vi "Main.vi"() -> ()   [LabVIEW 2020]
doc: "Use this template to build a simple state machine design pattern. Each state executes code and determines which state to transition to."
uses:
  controls/StateMachineVariables.ctl
  <vilib>/vision/Avi.llb/IMAQ AVI2 Refnum.ctl
  <vilib>/userDefined/High Color/IMAQdx.ctl
  <vilib>/vision/Deep Learning.llb/IMAQ DL Model Refnum.ctl
  <vilib>/vision/Image Controls.llb/IMAQ Image.ctl
  controls/State.ctl
panel:
  in  "Cluster":T1
  in  "Turn on the replay mode":bool=TRUE
  out "Replay mode":bool
  in  "?":T6(tab)
  in  "Camera Name":refnum<k21> caption="IMAQdx Session"
  out "fps cam":dbl
  out "height":u32
  out "width":u32
  in  "Start Frame Number":u32
  out "Actual frame":u32
  in  "Frame increment":i32=1
  in  "Video fps":u32=30
  in  "Video filename":string="test_moving2.avi"
  in  "Height":i32=1080
  in  "Width":i32=1920
  out "fps detection":dbl
  out "Distance":sgl(graph)
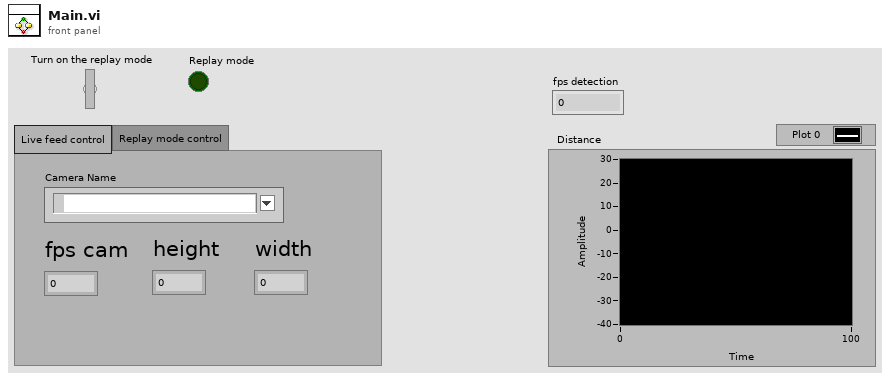
[diagram p1: front panel]
types:
  T1 = typedef "StateMachineVariables.ctl" = cluster{"AVI Refnum":T2, "Session ID":T3, "TensorFlow model refnum":T4, "Image refnum":T5, "VI path":path, "Horizontal distance":dbl, "Lateral distance":dbl, "Relative speed":dbl, "FPS":dbl}
  T2 = typedef "IMAQ AVI2 Refnum.ctl" = refnum<k20>
  T3 = typedef "IMAQdx.ctl" = refnum<k21>
  T4 = typedef "IMAQ DL Model Refnum.ctl" = refnum<k20>
  T5 = typedef "IMAQ Image.ctl" = refnum<image>
  T6 = enum32{"Live feed control", "Replay mode control"}
  T7 = typedef "State.ctl" = enum16{"Initialize VI path", "Initialize Video Session", "Initialize Cam session", "Initialize TensorFlow Model", "Initialize Image refnum", "Get video frame", "Get Cam frame", "Analyze image", "Update reaction space"}
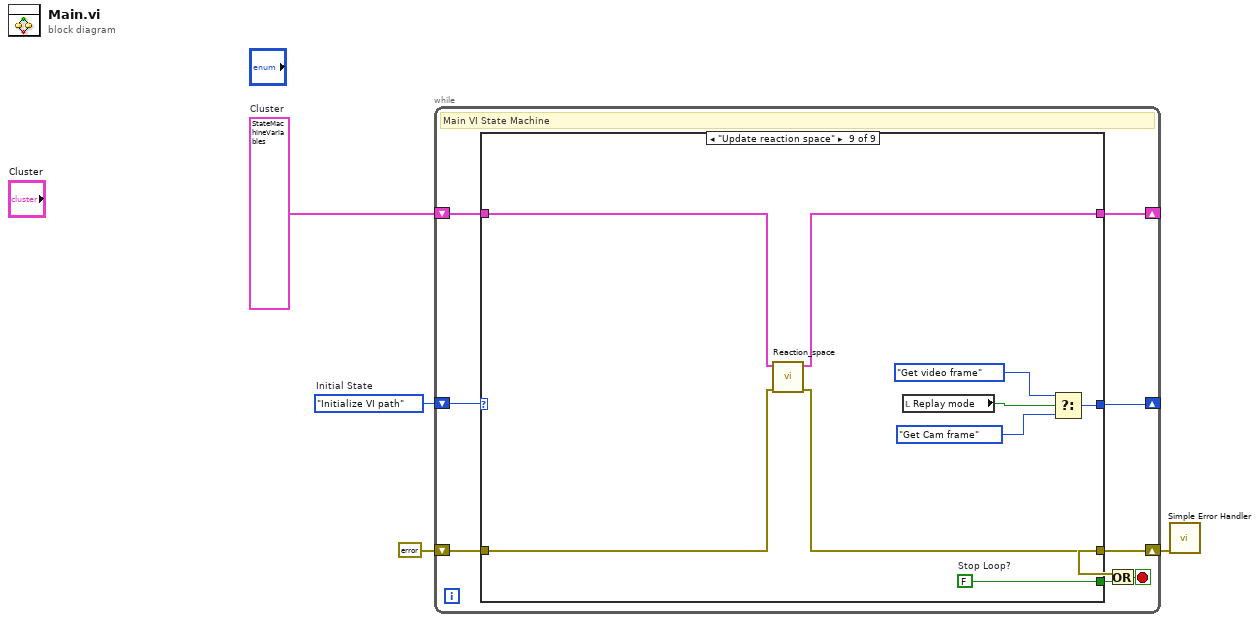
[diagram p0: block diagram]
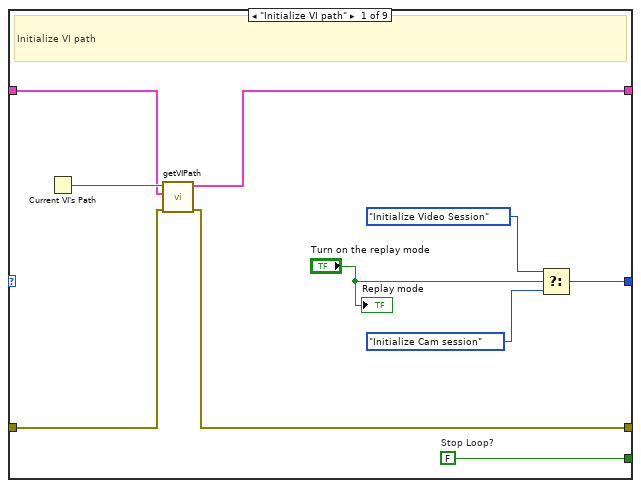
[diagram p2: hidden frame]
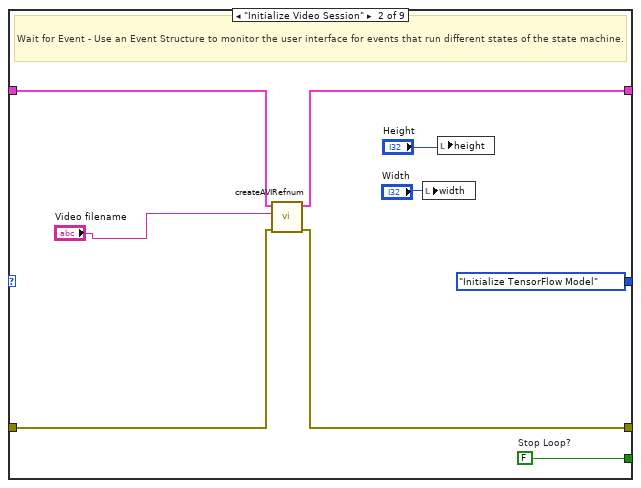
[diagram p3: hidden frame]
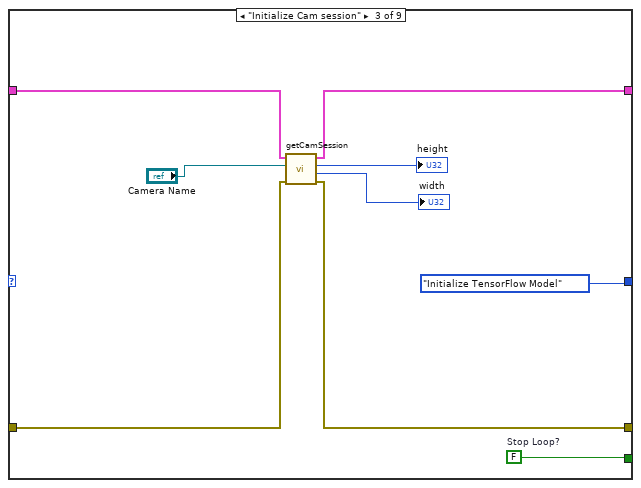
[diagram p4: hidden frame]
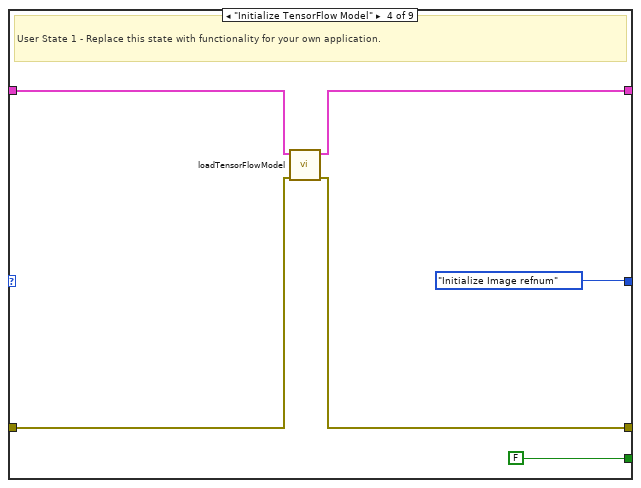
[diagram p5: hidden frame]
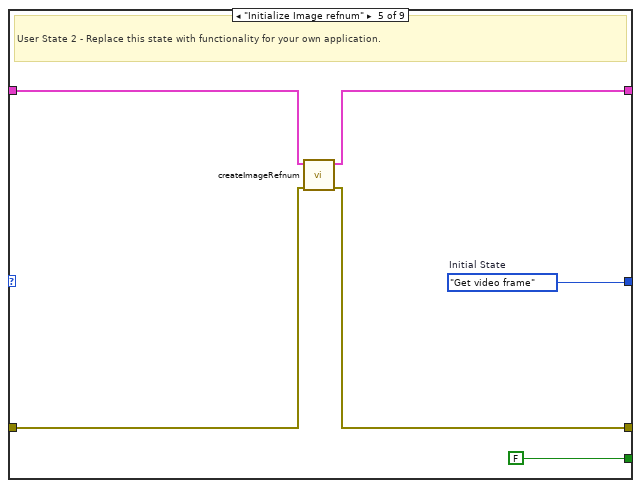
[diagram p6: hidden frame]
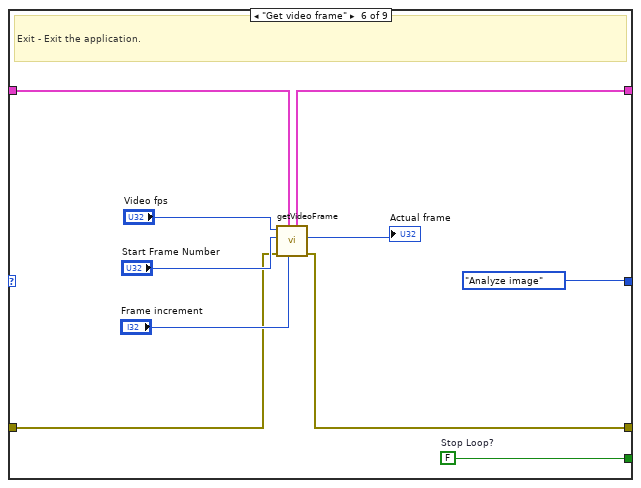
[diagram p7: hidden frame]
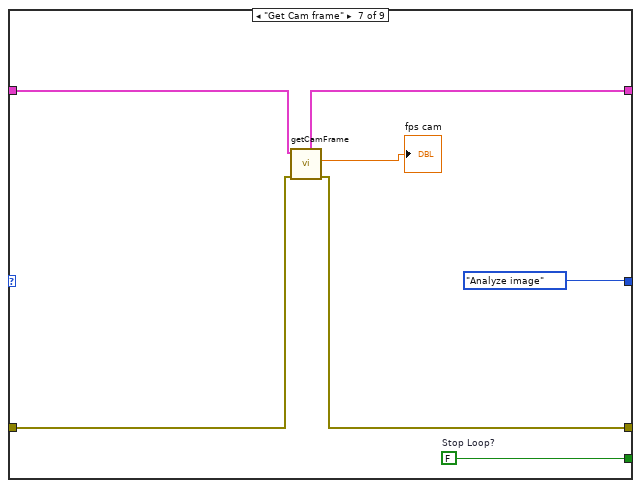
[diagram p8: hidden frame]
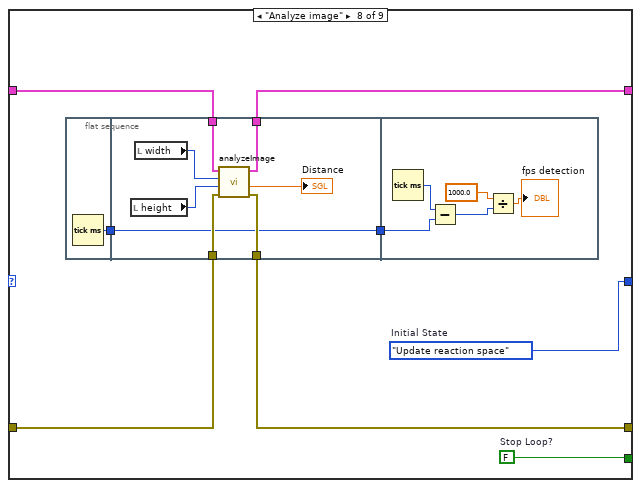
[diagram p9: hidden frame]
diagram:
  w2 = T1 {"AVI Refnum"=refnum, "Session ID"="", "TensorFlow model refnum"=refnum, "Image refnum"=refnum, "VI path"=path "", "Horizontal distance"=0.0, "Lateral distance"=0.0, "Relative speed"=0.0, "FPS"=0.0}  # Cluster
  w1 = State."Initialize VI path"  # Initial State
  n1 = while {
    shift-right: [w11] -> _
    shift-left: w2 -> [w12]
    shift-right: [w7] -> w3
    shift-left: errorcluster {"status"=FALSE, "code"=0, "source"=""} ("error constant") -> [w10]
    shift-right: [w6] -> _
    shift-left: w1 -> [w5]
    stop <- w8 stop-if-true
    # "Main VI State Machine"
    n2 = case shown="\"Update reaction space\"" w5 {
      tunnel: [w14 State."Initialize TensorFlow Model" State."Initialize TensorFlow Model" State."Initialize Image refnum" w49 State."Analyze image" State."Analyze image" w72 w93] -> w6
      tunnel: [w22 w31 w34 FALSE ("Stop Loop?") FALSE ("Stop Loop?") w62 w63 w73 w96] -> w9
      tunnel: w12 -> [w20 w26 w39 w44 w51 w57 w69 w77 w100]
      tunnel: [w19 w25 w38 w43 w50 w56 w68 w76 w99] -> w11
      tunnel: w10 -> [w17 w24 w37 w41 w47 w53 w66 w75 w98]
      tunnel: [w18 w23 w36 w42 w48 w54 w65 w74 w97] -> w7
      frame "Initialize VI path" {
        w22 = FALSE  # Stop Loop?
        # "Initialize VI path"
        n3 = Current VI's Path() -> (path=w21:path)
        n4 = call "getVIPath.vi"("error in"=w17, "Cluster in"=w20, "path"=w21) -> ("error out"=w18:errorcluster, "Cluster out"=w19:T1)  [unwired: 7 in]
        n5 = Select(t=State."Initialize Video Session", s="Turn on the replay mode", f=State."Initialize Cam session") -> (s? t:f=w14:T7)
        "Replay mode" <- "Turn on the replay mode"
      }
      frame "Initialize Video Session" {
        w31 = FALSE  # Stop Loop?
        # "Wait for Event - Use an Event Structure to monitor the user interface for events that run different states of the state machine."
        n6 = call "createAVIRefnum.vi"("error in"=w24, "Video filename"="Video filename", "Input cluster"=w26) -> ("error out"=w23:errorcluster, "Output cluster"=w25:T1)  [unwired: 7 in]
        n7 = local write "width"("Width") -> ()
        n8 = local write "height"("Height") -> ()
      }
      frame "Initialize Cam session" {
        w34 = FALSE  # Stop Loop?
        n9 = call "getCamSession.vi"("error in"=w37, "Camera name"="Camera Name", "Input cluster"=w39) -> ("error out"=w36:errorcluster, "Width"=→"width":u32, "Height"=→"height":u32, "Output cluster"=w38:T1)  [unwired: 5 in]
      }
      frame "Initialize TensorFlow Model" {
        # "User State 1 - Replace this state with functionality for your own application."
        n10 = call "loadTensorFlowModel.vi"("error in"=w41, "Input cluster"=w44) -> ("error out"=w42:errorcluster, "Output cluster"=w43:T1)  [unwired: 8 in]
      }
      frame "Initialize Image refnum" {
        w49 = State."Get video frame"  # Initial State
        # "User State 2 - Replace this state with functionality for your own application."
        n11 = call "createImageRefnum.vi"("error in"=w47, "Output cluster in"=w51) -> ("error out"=w48:errorcluster, "Output cluster out"=w50:T1)  [unwired: 8 in]
      }
      frame "Get video frame" {
        w62 = FALSE  # Stop Loop?
        # "Exit - Exit the application."
        n12 = call "getVideoFrame.vi"("Frame increment"="Frame increment", "Input cluster"=w57, "error in (no error)"=w53, "Start Frame Number"="Start Frame Number", "Video fps"="Video fps") -> ("error out"=w54:errorcluster, "Actual frame"=→"Actual frame":u32, "Iutput cluster"=w56:T1)  [unwired: 4 in]
      }
      frame "Get Cam frame" {
        w63 = FALSE  # Stop Loop?
        n13 = call "getCamFrame.vi"("error in (no error)"=w66, "Cluster"=w69) -> ("error out"=w65:errorcluster, "Acquired Frames per Second"=→"fps cam":dbl, "output cluster"=w68:T1)  [unwired: 7 in]
      }
      frame "Analyze image" {
        w73 = FALSE  # Stop Loop?
        w72 = State."Update reaction space"  # Initial State
        n14 = flat-sequence {
          tunnel: [w78] -> w71
          tunnel: w77 -> [w86]
          tunnel: [w85] -> w76
          tunnel: w75 -> [w81]
          tunnel: [w80] -> w74
          tunnel: w71 -> [w79]
          tunnel: [w79] -> w70
          tunnel: w70 -> [w88]
          frame #0 {
            n15 = Tick Count (ms)() -> (millisecond timer value=w78:u32)
          }
          frame #1 {
            n16 = local read "height"() -> (w82:u32)
            n17 = local read "width"() -> (w83:u32)
            n18 = call "analyzeImage.vi"("error in"=w81, "Height"=w82, "Width"=w83, "Input cluster"=w86) -> ("error out"=w80:errorcluster, "Output cluster"=w85:T1, "Distance"=→"Distance":sgl)  [unwired: 3 in, 2 out]
          }
          frame #2 {
            n19 = Tick Count (ms)() -> (millisecond timer value=w91:u32)
            n20 = Subtract(x=w91, y=w88) -> (x-y=w89:u32)
            n21 = Divide(x=1000.0, y=w89) -> (x/y=→"fps detection":dbl)
          }
        }
      }
      frame "Update reaction space" {
        w96 = FALSE  # Stop Loop?
        n22 = call "Reaction_space.vi"("error in"=w98, "Input cluster"=w100) -> ("error out"=w97:errorcluster, "Ouptut cluster"=w99:T1)  [unwired: 8 in]
        n23 = local read "Replay mode"() -> (w92:bool)
        n24 = Select(t=State."Get video frame", s=w92, f=State."Get Cam frame") -> (s? t:f=w93:T7)
      }
    }
    n25 = Or(x=w7, y=w9) -> (x .or. y?=w8:bool)
  }
  n26 = call <vilib>:"Simple Error Handler.vi"("error in (no error)"=w3) -> ()  [unwired: 4 in, 5 out]
